vi "Controls to Connector Pane.vi"(8 "error in (no error)":errorcluster, 9 "Wiring Rules":T1(array[ring]), 10 "Controls":refnum<vi>[](array[refnum]), 11 "vi ref in":refnum<vi>) -> (0 "error out":errorcluster, 3 "vi ref out":refnum<vi>)   [LabVIEW 2020, in "Message Maker.lvlib"]
uses:
  Message Maker.lvlib
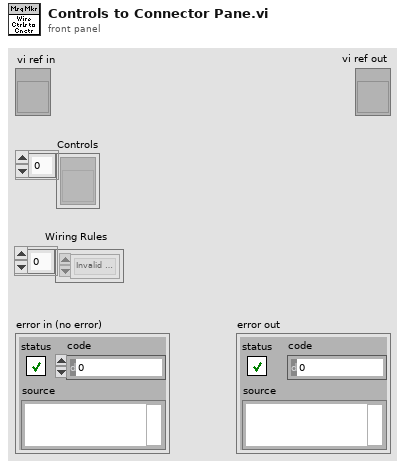
[diagram p1: front panel]
types:
  T1 = enum16{"Invalid Wire Rule", "Required", "Recommended", "Optional", "Dynamic Dispatch"}[]
  T2 = enum16{"Invalid Wire Rule", "Required", "Recommended", "Optional", "Dynamic Dispatch"}
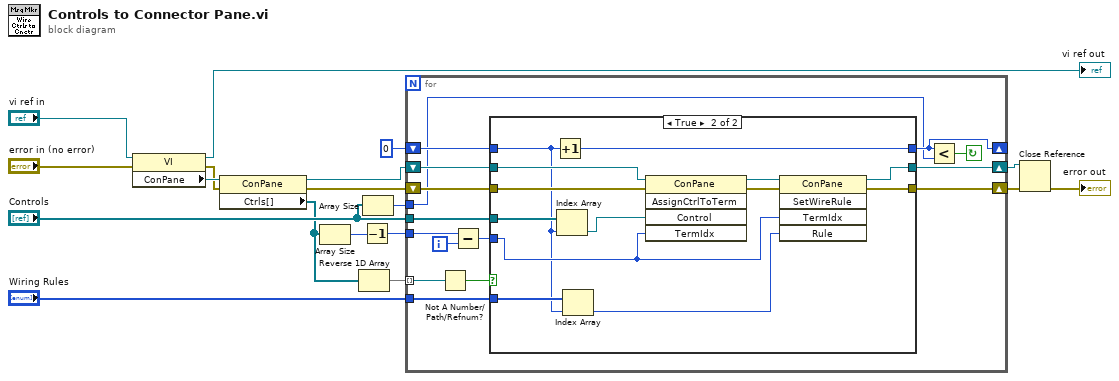
[diagram p0: block diagram]
diagram:
  n1 = property class="VI"(reference="vi ref in", error in="error in (no error)") -> (reference out=→"vi ref out":refnum<vi>, error out=w1:errorcluster, "ConPane"=w5:refnum<vi>)
  n2 = property class="ConPane"(reference=w5, error in=w1) -> (reference out=w9:refnum<vi>, error out=w10:errorcluster, "Ctrls[]"=w6:refnum<vi>[])
  n3 = Array Size(array=w6) -> (size(s)=w7:i32)
  n4 = Reverse 1D Array(array=w6) -> (reversed array=w2:refnum<vi>[])
  n5 = Decrement(x=w7) -> (x-1=w8:i32)
  n6 = Array Size(array="Controls") -> (size(s)=w17:i32)
  n7 = for {
    tunnel: w2 -> [w25] mode=indexing
    tunnel: w8 -> [w32]
    shift-right: [w30] -> w12
    shift-left: w9 -> [w31]
    shift-right: [w28] -> w11
    shift-left: w10 -> [w29]
    tunnel: "Controls" -> [w24]
    shift-right: [w21] -> _
    shift-left: 0 ("index") -> [w23]
    tunnel: w17 -> [w20]
    tunnel: "Wiring Rules" -> [w19]
    i -> [w33]
    stop <- w22 continue-if-true
    n8 = Not A Number/Path/Refnum?(number/path/refnum=w25) -> (NaN/Path/Refnum?=w27:bool)
    n9 = Subtract(x=w32, y=w33) -> (x-y=w26:i32)
    n10 = case shown="True" w27 {
      tunnel: w31 -> [w36 w49]
      tunnel: [w36 w43] -> w30
      tunnel: w29 -> [w35 w48]
      tunnel: [w35 w44] -> w28
      tunnel: w26 -> [_ w42]
      tunnel: w24 -> [_ w39]
      tunnel: w23 -> [w34 w38]
      tunnel: [w34 w47] -> w21
      tunnel: w19 -> [_ w41]
      frame False {
      }
      frame True {
        n11 = Increment(x=w38) -> (x+1=w47:i32)
        n12 = Index Array(array=w39, index=w38) -> (element=w37:refnum<vi>)
        n13 = Index Array(array=w41, index=w38) -> (element=w40:T2)
        n14 = invoke class="ConPane" method="AssignCtrlToTerm"(reference=w49, error in=w48, "Control"=w37, "TermIdx"=w42) -> (reference out=w46:refnum<vi>, error out=w45:errorcluster)  [unwired: 1 in, 3 out]
        n15 = invoke class="ConPane" method="SetWireRule"(reference=w46, error in=w45, "TermIdx"=w42, "Rule"=w40) -> (reference out=w43:refnum<vi>, error out=w44:errorcluster)  [unwired: 1 in, 3 out]
      }
    }
    n16 = Less?(x=w21, y=w20) -> (x < y?=w22:bool)
  }
  n17 = Close Reference(reference=w12, error in (no error)=w11) -> (error out=→"error out":errorcluster)
